vi "总磷氨氮插入数据.vi"(0 "database":string, 1 "data":T2 {"单位" items=["ug/L", "mg/L", "ppm", "mg/m3", "cm", "ppb", "ug/m3", "%", "nmol/mol", "umol/mol", "MPN/L", "MPN/100ml", "ng/m3", "NTU", "无量纲", "ms/cm", "us/cm"]}, 3 "SN":string, 5 "table":string, 7 "测量模式":T1(ring)=enum."水样测试", 9 "数据标记表":string(combo)="N", 11 "error in (no error)":errorcluster) -> (15 "error out":errorcluster)   [LabVIEW 2016, in "斯坦道氨氮.lvlib"]
uses:
  <vilib>/Utility/sysdir.llb/System Directory Type.ctl
  <vilib>/addons/database/Connection.llb/DB Tools Open Connec (String).vi
  <vilib>/addons/database/Connection.llb/Conn Execute.vi
  <vilib>/addons/database/Recordset.llb/Rec Destroy - Connection.vi
  <vilib>/addons/database/Recordset.llb/Rec Fetch Recordset Data (R).vi
  <vilib>/addons/database/NI_Database_API.lvlib
panel:
  out "为空？":bool
  out "recordset data":variant[][](array[variant])
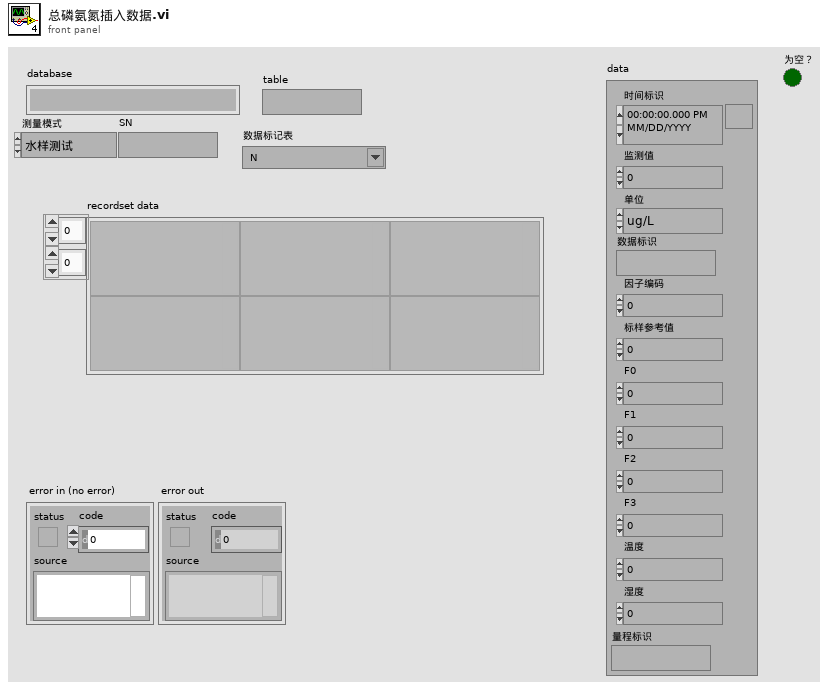
[diagram p1: front panel]
types:
  T1 = enum16{"维护数据", "水样测试", "标样核查", "零点核查", "跨度核查", "空白测试", "平行样测试", "加标回收", "空白校准", "标样校准", "初始化（清洗）"}
  T2 = cluster{"时间标识":timestamp, "监测值":sgl, "单位":u16, "数据标识":string, "因子编码":u32, "标样参考值":sgl, "F0":sgl, "F1":sgl, "F2":sgl, "F3":sgl, "温度":sgl, "湿度":sgl, "量程标识":string}
  T3 = typedef "System Directory Type.ctl" = i32
  T4 = typedef "NI_Database_API.lvlib/Conn ObjectReference.ctl" = refnum<k1>
  T5 = typedef "NI_Database_API.lvlib/Rec ObjectReference.ctl" = refnum<k1>
  T6 = cluster{"时间标识":timestamp, "测量模式":string, "数据类型":string, "监测值":sgl, "单位":string, "数据标识":string, "因子编码":string, "标样参考值":sgl, "F0":sgl, "F1":sgl, "F2":sgl, "F3":sgl, "温度":sgl, "湿度":sgl, "量程标识":string, "SN":string}
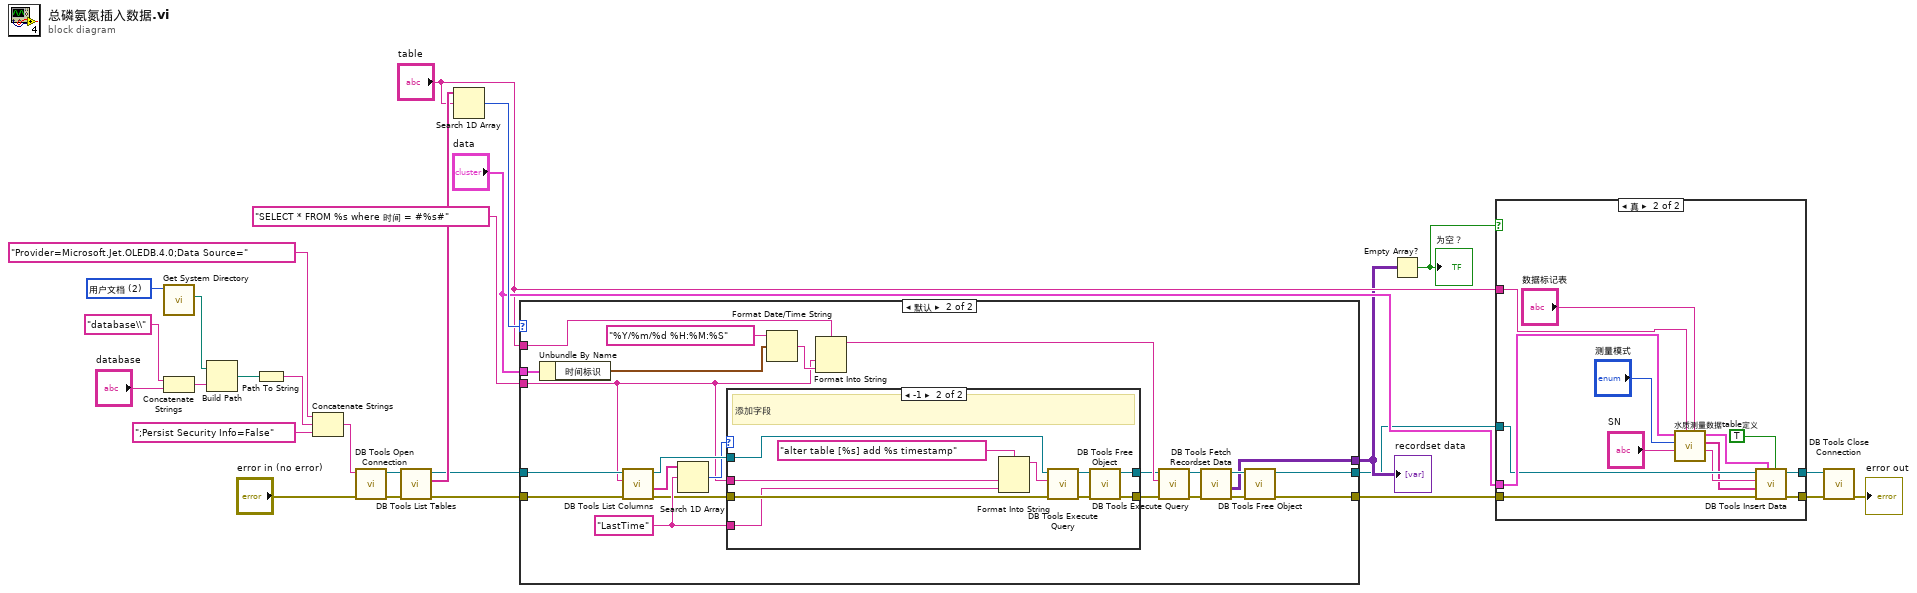
[diagram p0: block diagram]
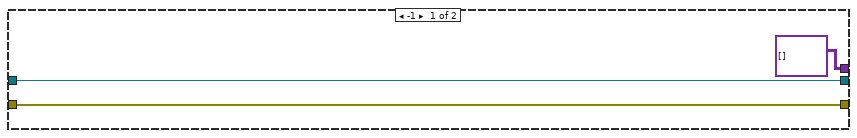
[diagram p2: hidden frame]
diagram:
  w26 = T3 2 items=["用户目录"=0, "用户桌面"=1, "用户文档"=2, "用户应用程序数据"=3, "用户设置"=4, "用户临时目录"=5, "公共文档"=6, "公共应用程序数据"=7, "公共设置"=8, "公共缓存"=13, "系统核心库"=9, "系统安装库"=10, "应用程序文件"=11, "启动盘根目录"=12] ("system directory type")
  n1 = call <vilib>:"Get System Directory.vi"("system directory type"=w26) -> ("system directory"=w24:path)  [unwired: 10 in]
  n2 = Concatenate Strings("database\\" ("condition"), "database") -> (w18:string)
  n3 = Build Path(base path=w24, name or relative path=w18) -> (appended path=w23:path)
  n4 = Path To String(path=w23) -> (string=w22:string)
  n5 = Concatenate Strings("Provider=Microsoft.Jet.OLEDB.4.0;Data Source=" ("condition"), w22, ";Persist Security Info=False" ("condition")) -> (w20:string)
  n6 = call-poly <vilib>:"DB Tools Open Connection.vi"("error in (no error)"="error in (no error)", "connection information"=w20) -> ("error out"=w16:errorcluster, "connection reference"=w17:T4)  [unwired: 6 in]
  n7 = call <vilib>:"DB Tools List Tables.vi"("error in (no error)"=w16, "connection reference"=w17) -> ("error out"=w4:errorcluster, "tables"=w15:string[], "connection reference out"=w5:T4)  [unwired: 3 in]
  n8 = Search 1D Array(1D array=w15, element="table") -> (index of element=w9:i32)  [unwired: 1 in]
  n9 = case shown="默认" w9 {
    tunnel: [variant[][] [] ("recordset data") w31] -> w3
    tunnel: [w30 w49] -> w2
    tunnel: [w29 w48] -> w1
    tunnel: w5 -> [w30 w34]
    tunnel: w4 -> [w29 w33]
    tunnel: "SELECT * FROM %s where 时间 = #%s#" ("格式字符串") -> [_ w32]
    tunnel: "table" -> [_ w47]
    tunnel: "data" -> [_ w42]
    frame -1 {
    }
    frame Default {
      w40 = "LastTime" ("元素")
      n10 = Unbundle By Name(w42) -> ("时间标识"=w45:timestamp)
      n11 = call <vilib>:"DB Tools List Columns.vi"("error in (no error)"=w33, "table"=w32, "connection reference"=w34) -> ("error out"=w38:errorcluster, "columns"=w39:string[], "connection reference out"=w41:T4)  [unwired: 1 in, 1 out]
      n12 = Search 1D Array(1D array=w39, element=w40) -> (index of element=w37:i32)  [unwired: 1 in]
      n13 = case shown="-1" w37 {
        tunnel: w41 -> [w55 w63]
        tunnel: w38 -> [w54 w62]
        tunnel: w40 -> [_ w60]
        tunnel: [w55 w58] -> w36
        tunnel: [w54 w57] -> w35
        tunnel: w32 -> [_ w56]
        frame 0, Default {
        }
        frame -1 {
          # "添加字段"
          n14 = Format Into String(format string="alter table [%s] add %s timestamp", w56, w60) -> (resulting string=w59:string)  [unwired: 2 in, 1 out]
          n15 = call-poly <vilib>:"DB Tools Execute Query.vi"("error in (no error)"=w62, "SQL query"=w59, "connection reference"=w63) -> ("error out"=w64:errorcluster, "recordset reference"=w65:T5)  [unwired: 5 in]
          n16 = call-poly <vilib>:"DB Tools Free Object.vi"("error in (no error)"=w64, "recordset reference"=w65) -> ("error out"=w57:errorcluster, "connection reference"=w58:T4)  [unwired: 8 in]
        }
      }
      n17 = Format Date/Time String(time format string (%c)="%Y/%m/%d %H:%M:%S" ("时间格式字符串(%c)"), seconds (now)=w45) -> (date/time string=w43:string)  [unwired: 1 in]
      n18 = Format Into String(format string=w47, w32, w43) -> (resulting string=w46:string)  [unwired: 2 in, 1 out]
      n19 = call-poly <vilib>:"DB Tools Execute Query.vi"("error in (no error)"=w35, "SQL query"=w46, "connection reference"=w36) -> ("error out"=w50:errorcluster, "recordset reference"=w53:T5)  [unwired: 5 in]
      n20 = call-poly <vilib>:"DB Tools Fetch Recordset Data.vi"("error in (no error)"=w50, "recordset reference"=w53) -> ("error out"=w51:errorcluster, "recordset data"=w31:variant[][], "recordset reference out"=w52:T5)  [unwired: 3 in]
      n21 = call-poly <vilib>:"DB Tools Free Object.vi"("error in (no error)"=w51, "recordset reference"=w52) -> ("error out"=w48:errorcluster, "connection reference"=w49:T4)  [unwired: 8 in]
    }
  }
  "recordset data" <- w3
  n22 = Empty Array?(array=w3) -> (empty?=w13:bool)
  "为空？" <- w13
  n23 = case shown="真" w13 {
    tunnel: "table" -> [_ w80]
    tunnel: "data" -> [_ w79]
    tunnel: w1 -> [w66 w77]
    tunnel: w2 -> [w67 w76]
    tunnel: [w67 w71] -> w12
    tunnel: [w66 w70] -> w11
    frame False {
    }
    frame True {
      n24 = call "水质测量数据table定义.vi"("数据标记表"="数据标记表", "table 输入"=w80, "SN"="SN", "测量模式"="测量模式", "data"=w79) -> ("table 输出"=w73:string, "columns"=w72:string[], "data输出"=w75:T6)  [unwired: 4 in]
      n25 = call <vilib>:"DB Tools Insert Data.vi"("create table? (F)"=TRUE, "data"=w75, "error in (no error)"=w77, "columns"=w72, "table"=w73, "connection reference"=w76) -> ("error out"=w70:errorcluster, "connection reference out"=w71:T4)  [unwired: 4 in]
    }
  }
  n26 = call <vilib>:"DB Tools Close Connection.vi"("error in (no error)"=w11, "connection reference"=w12) -> ("error out"=→"error out":errorcluster)  [unwired: 5 in]
